vi "mWmotor_get_movestatus.vi"(8 "error in (no error)":errorcluster, 10 "milliseconds to wait":u32=100, 11 "VISA resource name":refnum<visa-resource-name>) -> (0 "error out":errorcluster, 2 "VISA resource name out":refnum<visa-resource-name>, 3 "Boolean":bool)   [LabVIEW 2019]
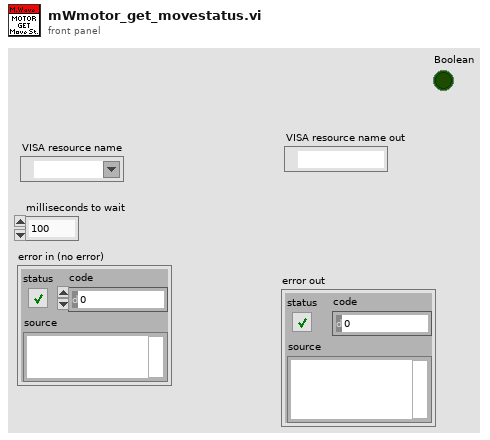
[diagram p1: front panel]
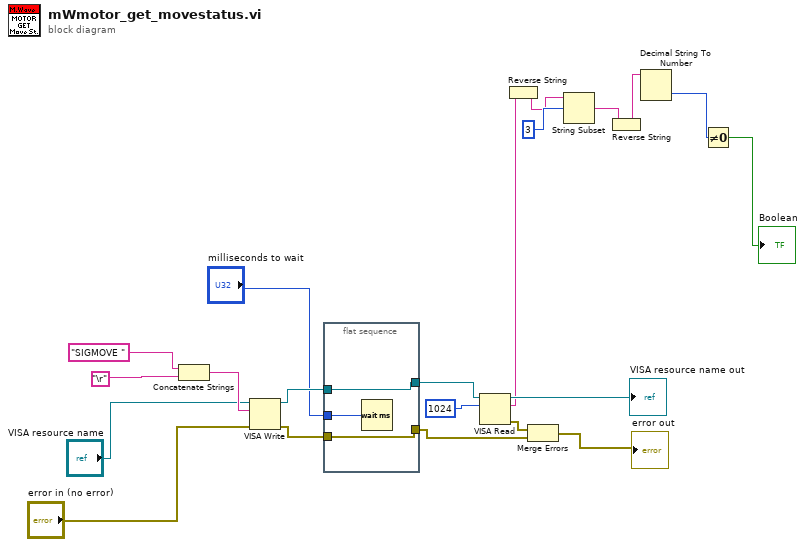
[diagram p0: block diagram]
diagram:
  n1 = Concatenate Strings("SIGMOVE " ("string"), "\r") -> (w21:string)
  n2 = VISA Write(VISA resource name="VISA resource name", write buffer=w21, error in (no error)="error in (no error)") -> (VISA resource name out=w16:refnum<visa-resource-name>, error out=w17:errorcluster)  [unwired: 1 out]
  n3 = flat-sequence {
    tunnel: [w24] -> w10
    tunnel: w17 -> [w24]
    tunnel: [w23] -> w15
    tunnel: w16 -> [w23]
    tunnel: "milliseconds to wait" -> [w22]
    frame #0 {
      n4 = Wait (ms)(milliseconds to wait=w22) -> ()  [unwired: 1 out]
    }
  }
  n5 = VISA Read(VISA resource name=w15, byte count=u32 1024) -> (VISA resource name out=→"VISA resource name out":refnum<visa-resource-name>, read buffer=w1:string, error out=w8:errorcluster)  [unwired: 1 in, 1 out]
  n6 = Reverse String(1:w1) -> (0:w6:string)
  n7 = Merge Errors(w8, w10) -> (→"error out":errorcluster)
  n8 = String Subset(string=w6, offset (0)=3) -> (substring=w5:string)  [unwired: 1 in]
  n9 = Reverse String(1:w5) -> (0:w4:string)
  n10 = Decimal String To Number(string=w4) -> (number=w3:i32)  [unwired: 2 in, 1 out]
  n11 = Not Equal To 0?(x=w3) -> (x != 0?=→"Boolean":bool)
